vi "p10y3.vi"() -> ()   [LabVIEW 2020]
uses:
  <vilib>/sound2/lvsound2.llb/Sound Data Format.ctl
  <vilib>/sound2/lvsound2.llb/Sound Output Set Volume (Single).vi
  <vilib>/sound2/lvsound2.llb/Sound Input Read (DBL).vi
  <vilib>/sound2/lvsound2.llb/Sound Output Write (DBL).vi
  <vilib>/express/express analysis/Spectral/Block/exnSpectralBlock spectral measurements peak poly.vi
  <vilib>/express/express analysis/Spectral/Block/exnSpectralBlock spectral measurements peak DDT.vi
  <vilib>/express/express analysis/Spectral/Block/exnSpectralBlock spectral measurements peak array WFM.vi
  <vilib>/express/express analysis/Spectral/XNode/ExpressSpectralMeasurementsBlockNode.xnode
panel:
  in  "volume":dbl=100.0
  out "FILTER FFT":dynamicdata(graph)
  out "AEG FILTER":dynamicdata(graph)
  out "Originaal FFT":cluster{"f0":dbl, "df":dbl, "magnitude":dbl[]}[](graph)
  out "AEG ORIKAS":waveform(dbl)[](graph)
  in  "FILTER/ORIGINAAL":bool
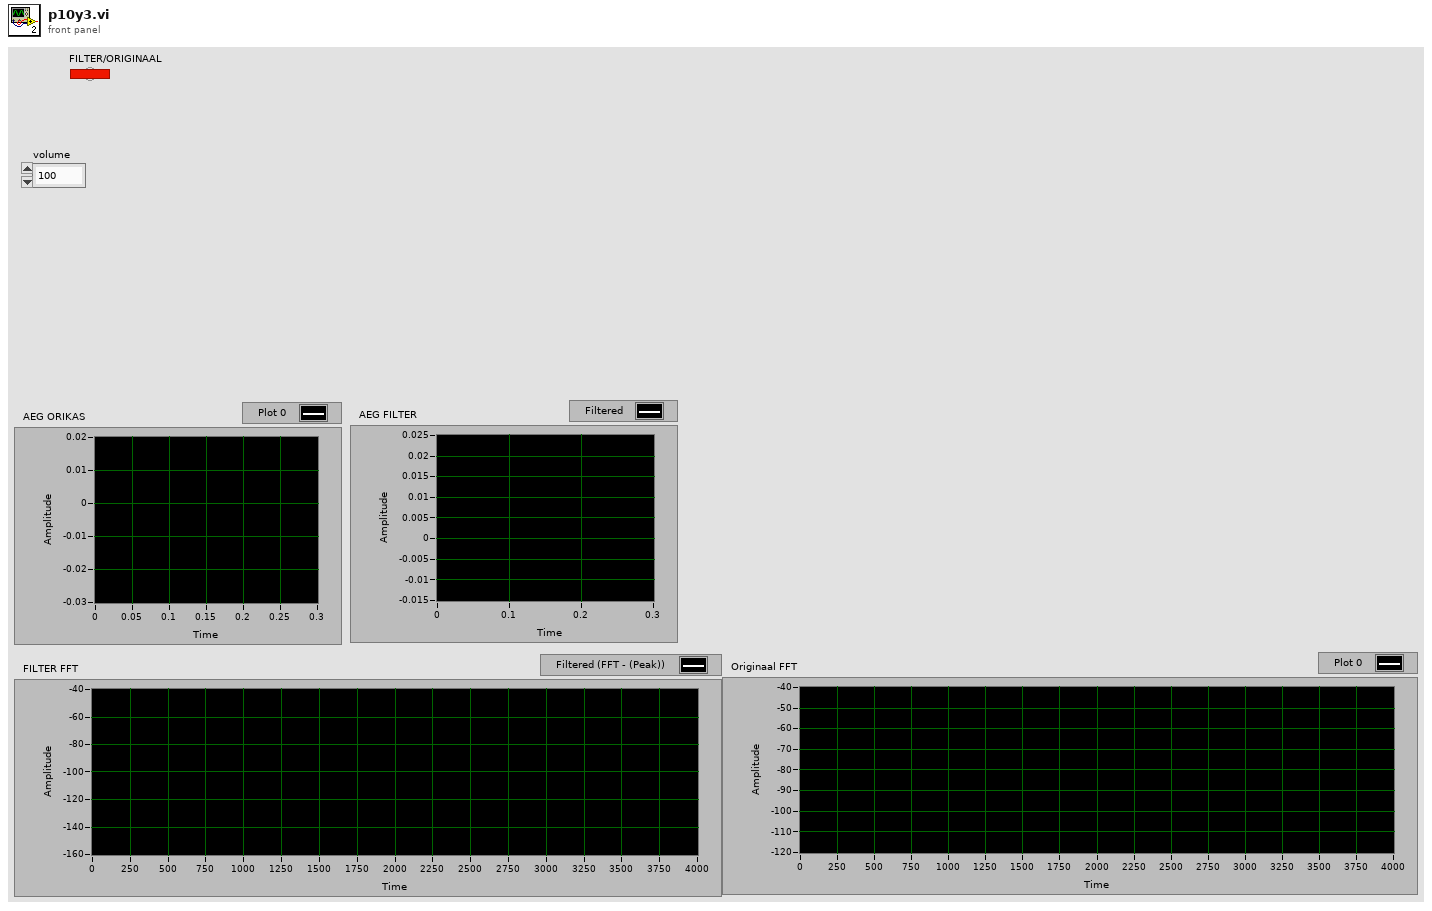
[diagram p1: front panel]
types:
  T1 = typedef "Sound Data Format.ctl" = cluster{"sample rate (S/s)":dbl, "number of channels":i32, "bits per sample":i32}
  T2 = typedef "Sound Input Task ID.ctl" = u32
  T3 = typedef "Sound Output Task ID.ctl" = u32
  T4 = cluster{"averaging mode":u16, "weighting mode":u16, "number of averages":u32}
  T5 = cluster{"dB On (F)":bool, "unwrap phase (F)":bool, "convert to degree (F)":bool}
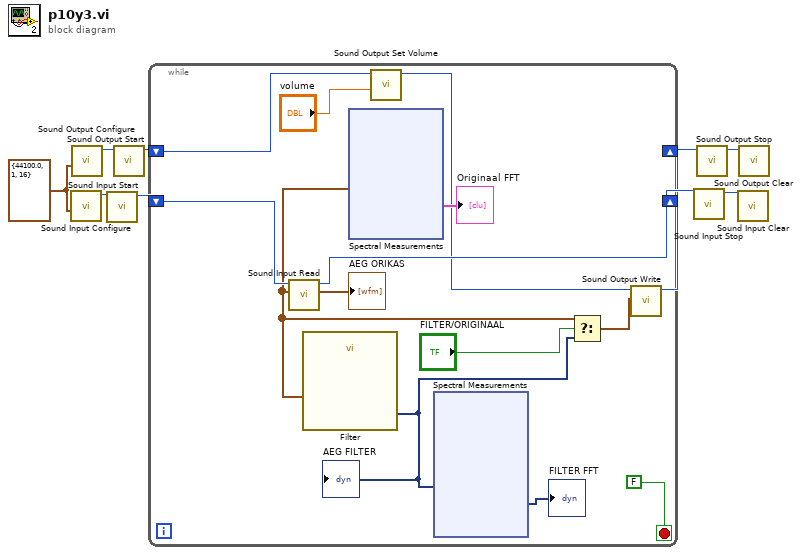
[diagram p0: block diagram]
diagram:
  w9 = T1 {"sample rate (S/s)"=44100.0, "number of channels"=1, "bits per sample"=16} ("sound format")
  n1 = call <vilib>:"Sound Input Configure.vi"("sound format"=w9) -> ("task ID"=w8:T2)  [unwired: 9 in, 1 out]
  n2 = call <vilib>:"Sound Output Configure.vi"("sound format"=w9) -> ("task ID"=w4:T3)  [unwired: 9 in, 1 out]
  n3 = call <vilib>:"Sound Input Start.vi"("task ID"=w8) -> ("task ID out"=w7:T2)  [unwired: 9 in, 1 out]
  n4 = call <vilib>:"Sound Output Start.vi"("task ID"=w4) -> ("task ID out"=w3:T3)  [unwired: 9 in, 1 out]
  n5 = while {
    shift-right: [w21] -> w6
    shift-left: w7 -> [w22]
    shift-right: [w12] -> w1
    shift-left: w3 -> [w20]
    stop <- FALSE stop-if-true
    n6 = call-poly <vilib>:"Sound Input Read.vi"("task ID"=w22) -> ("data"=w16:waveform(dbl)[], "task ID out"=w21:T2)  [unwired: 8 in, 1 out]
    "AEG ORIKAS" <- w16
    n7 = call "Filter"("Signal"=w16) -> ("Filtered Signal"=w17:dynamicdata)  [unwired: 9 in, 1 out]
    "AEG FILTER" <- w17
    n8 = xnode "Spectral Measurements"("Signals"=w16) -> ("FFT - (Peak)"=→"Originaal FFT":cluster{"f0":dbl, "df":dbl, "magnitude":dbl[]}[])  [unwired: 1 in, 2 out]
    n9 = call-poly <vilib>:"Sound Output Set Volume.vi"("volume"="volume", "task ID"=w20) -> ("task ID out"=w13:T3)  [unwired: 8 in, 1 out]
    n10 = xnode "Spectral Measurements"("Signals"=w17) -> ("FFT - (Peak)"=→"FILTER FFT":dynamicdata)  [unwired: 1 in, 2 out]
    n11 = Select(t=w16, s="FILTER/ORIGINAAL", f=w17) -> (s? t:f=w14:waveform(dbl)[])
    n12 = call-poly <vilib>:"Sound Output Write.vi"("data"=w14, "task ID"=w13) -> ("task ID out"=w12:T3)  [unwired: 8 in, 1 out]
  }
  n13 = call <vilib>:"Sound Input Stop.vi"("task ID"=w6) -> ("task ID out"=w5:T2)  [unwired: 9 in, 1 out]
  n14 = call <vilib>:"Sound Output Stop.vi"("task ID"=w1) -> ("task ID out"=w2:T3)  [unwired: 9 in, 1 out]
  n15 = call <vilib>:"Sound Input Clear.vi"("task ID"=w5) -> ()  [unwired: 10 in, 1 out]
  n16 = call <vilib>:"Sound Output Clear.vi"("task ID"=w2) -> ()  [unwired: 10 in, 1 out]
